vi "Install Simulated Device.vi"() -> (0 "error out":errorcluster, 3 "Device Name":tag="SMO-Sim")   [LabVIEW 2016, in "DAQmx-AI.lvclass"]
uses:
  DAQmx-AI.lvclass
  <vilib>/nisyscfg/nisyscfg.lvlib
panel:
  # "This VI installs the Simulated SMO Device from the NCE file located in the same folder"
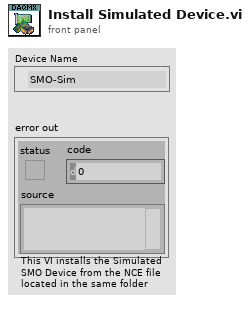
[diagram p1: front panel]
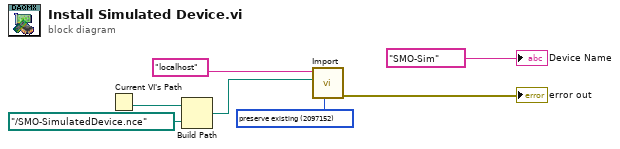
[diagram p0: block diagram]
diagram:
  w5 = u32 2097152 items=["merge"=0, "replace all"=1048576, "preserve existing"=2097152] ("Import Mode")
  n1 = Current VI's Path() -> (path=w4:path)
  n2 = Build Path(base path=w4, name or relative path=path "../SMO-SimulatedDevice.nce") -> (appended path=w2:path)
  n3 = call <vilib>:"Import.vi"("Import Mode"=w5, "Source File"=w2, "Session in"="localhost") -> ("error out"=→"error out":errorcluster)  [unwired: 6 in, 2 out]
  "Device Name" <- tag "SMO-Sim" ("ActiveDev")
